vi "Create Reply Messages.vi"(10 "Replies":u8[](array[numeric])) -> (2 "String Replies":string[](array[string]))   [LabVIEW 2024]
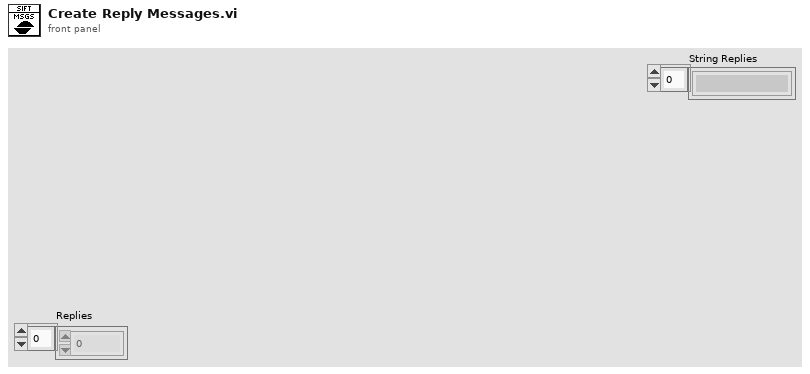
[diagram p1: front panel]
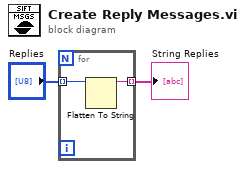
[diagram p0: block diagram]
diagram:
  n1 = for {
    tunnel: "Replies" -> [w4] mode=indexing
    tunnel: [w3] -> w1 mode=indexing
    n2 = Flatten To String(anything=w4) -> (data string=w3:string)  [unwired: 3 in, 2 out]
  }
  "String Replies" <- w1
